vi "MAT_TestingVI.vi"() -> ()   [LabVIEW 2024]
uses:
  Subs/miDataType.ctl
panel:
  out "unsigned byte array":u8[](array[numeric])
  out "dimensions":i32[](array[numeric])
  out "Arrays same?":bool
  out "Matrix":T2
  out "Waveform Graph":i16[](graph)
  out "unsigned byte array 2":u8[](array[numeric])
  out "mine":u8[](array[numeric]) format="%.0b"
  out "Bytes same?":bool
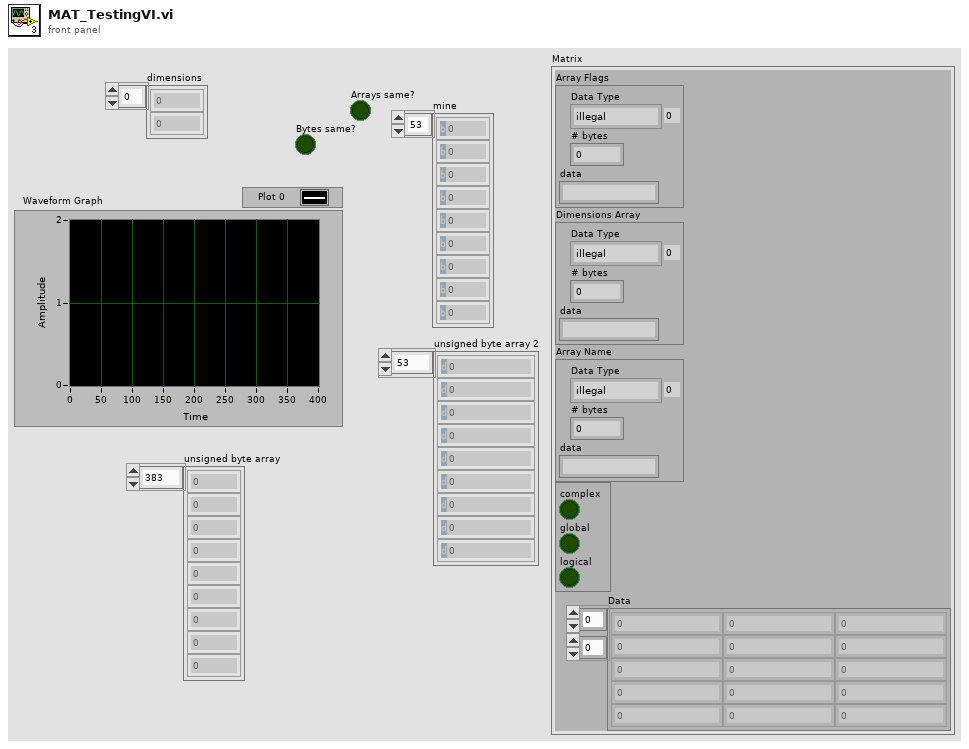
[diagram p1: front panel]
types:
  T1 = typedef "miDataType.ctl" = enum16{"illegal", "miINT8", "miUINT8", "miINT16", "miUINT16", "miINT32", "miUINT32", "miSINGLE", "--", "miDOUBLE", "---", "----", "miINT64", "miUINT64", "miMATRIX", "miCOMPRESSED", "miUTF8", "miUTF16", "miUTF32", "udefined"}
  T2 = cluster{"Array Flags":cluster{"Data Type":T1, "# bytes":u32, "data":string}, "Dimensions Array":cluster{"Data Type":T1, "# bytes":u32, "data":string}, "Array Name":cluster{"Data Type":T1, "# bytes":u32, "data":string}, cluster{"complex":bool, "global":bool, "logical":bool}, "Data":dbl[][]}
  T3 = enum16{"big-endian, network order", "native, host order", "little-endian"}
  T4 = cluster{"Data Type":T1, "# bytes":u32, "data":string}
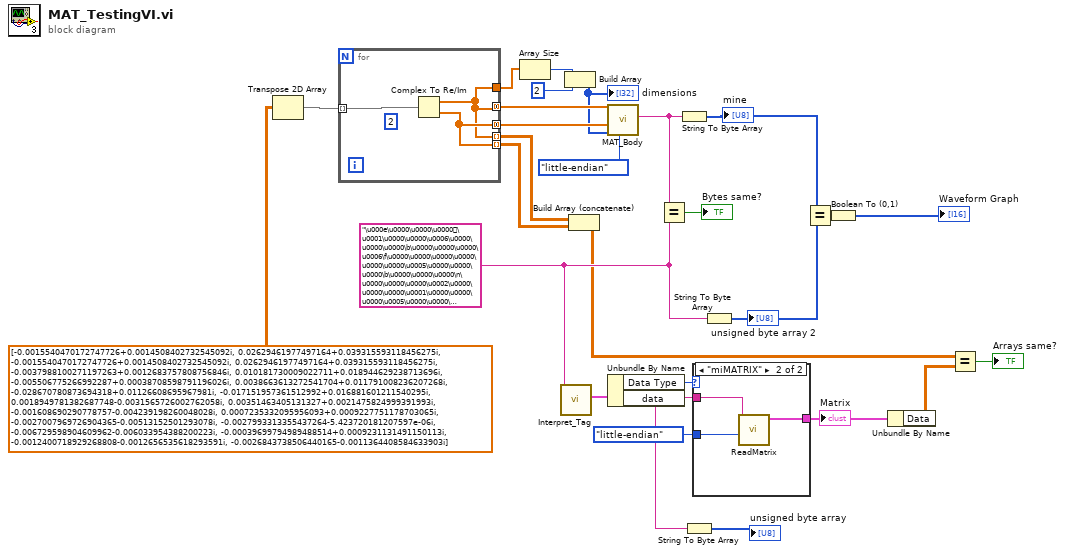
[diagram p0: block diagram]
diagram:
  w17 = "\u000e\u0000\u0000\u0000\u0001\u0000\u0000\u0006\u0000\u0000\u0000\b\u0000\u0000\u0000\u0006\f\u0000\u0000\u0000\u0000\u0000\u0000\u0005\u0000\u0000\u0000\b\u0000\u0000\u0000\n\u0000\u0000\u0000\u0002\u0000\u0000\u0000\u0001\u0000\u0000\u0000\u0005\u0000\u0000\u0000yspec\u0000\u0000\u0000\t\u0000\u0000\u0000 \u0000\u0000\u0000«fG%vY¿«fG%vY¿h÷®\u001eo¿·ÙºEv¿¸-Ðß[¿ö\u0019ZH\u001d\f_?ûæ\f\fV[Z¿\u0007wUû\u001ff¿S2^ó~{¿Hc\u000e=QT¿Ê\u001eú\u000fúì?Ê\u001eú\u000fúì?×^>«(Ú?(ûîX¬o?#h¸_H¿3|ÙÉ¸Êl?¸'¼oµG?²-îf¿J×\u001c6\u0004:¿þÂ<ýe¿\t\u0000\u0000\u0000 \u0000\u0000\u0000wLáCÅW?wLáCÅW?ûÝ\u001fôÇT?P¨¨9^9?Ì ]¬\u0012?­½\u0002ÐÛi¿ôí5\u001e\u001f]q¿q\r¿AË\u0004u¿\u0018½4L\u000f·x¿_ëý)¼T¿7NUe,!¤?7NUe,!¤?Í{\u000f8f?ÀL\u0017Vâ%?Cn\u0014iI?'SIÎa?ÓÛõyÌ<N?1ìÙ¬¿Ö¾\\9d¢?N?SA\u0014R¿"
  n1 = Transpose 2D Array(2D array=cdb[][] [[-0.0015540470172747726+0.0014508402732545092i, 0.02629461977497164+0.039315593118456275i], [-0.0015540470172747726+0.0014508402732545092i, 0.02629461977497164+0.039315593118456275i], [-0.0037988100271197263+0.0012683757808756846i, 0.010181730009022711+0.018944629238713696i], [-0.005506775266992287+0.00038708598791196026i, 0.0038663613272541704+0.011791008236207268i], [-0.028670780873694318+0.01126608695967981i, -0.017151957361512992+0.016881601211540295i], [0.0018949781382687748-0.0031565726002762058i, 0.00351463405131327+0.0021475824999391993i], [-0.001608690290778757-0.004239198260048028i, 0.0007235332095956093+0.0009227751178703065i], [-0.0027007969726904365-0.00513152501293078i, -0.0027993313355437264-5.423720181207597e-06i], [-0.006729598904609962-0.006033954388200223i, -0.00039699794989488514+0.0009231131491150113i], [-0.0012400718929268808-0.0012656535618293591i, -0.0026843738506440165-0.0011364408584633903i]] ("complex")) -> (transposed array=w20:cdb[][])
  n2 = for {
    tunnel: w20 -> [w30] mode=indexing
    tunnel: [w28] -> w11 mode=concatenating
    tunnel: [w29] -> w14 mode=concatenating
    tunnel: [w28] -> w7 mode=indexing
    tunnel: [w29] -> w6 mode=indexing
    tunnel: [w28] -> w8
    (unwired) 2 ("index")
    n3 = Complex To Re/Im(x + iy=w30) -> (x=w28:dbl[], y=w29:dbl[])
  }
  n4 = Array Size(array=w8) -> (size(s)=w3:i32)
  n5 = call "Interpret_Tag.vi"("String in"=w17) -> ("Tag"=w19:T4)  [unwired: 8 in, 2 out]
  n6 = Build Array(w3, 2 ("index")) -> (w1:i32[])
  "dimensions" <- w1
  n7 = Build Array (concatenate)(w7, w6) -> (w13:dbl[][])
  n8 = call "MAT_Body.vi"("byte order"=T3."little-endian", "Dimensions"=w1, "Imag"=w14, "Real"=w11) -> ("String Out"=w25:string)  [unwired: 6 in, 1 out]
  n9 = Unbundle By Name(w19) -> ("Data Type"=w18:T1, "data"=w4:string)
  n10 = Equal?(x=w25, y=w17) -> (x = y?=→"Bytes same?":bool)
  n11 = String To Byte Array(string=w25) -> (unsigned byte array=w24:u8[])
  "mine" <- w24
  n12 = String To Byte Array(string=w4) -> (unsigned byte array=→"unsigned byte array":u8[])
  n13 = case shown="\"miMATRIX\"" w18 {
    tunnel: w4 -> [_ w33]
    tunnel: [_ w31] -> w15
    tunnel: T3."little-endian" ("Endian") -> [_ w32]
    frame Default {
    }
    frame "miMATRIX" {
      n14 = call "ReadMatrix.vi"("byte order"=w32, "String in"=w33) -> ("Matrix"=w31:T2)  [unwired: 6 in, 3 out]
    }
  }
  "Matrix" <- w15
  n15 = String To Byte Array(string=w17) -> (unsigned byte array=w21:u8[])
  "unsigned byte array 2" <- w21
  n16 = Equal?(x=w24, y=w21) -> (x = y?=w23:bool[])
  n17 = Boolean To (0,1)(Boolean=w23) -> (0, 1=→"Waveform Graph":i16[])
  n18 = Unbundle By Name(w15) -> ("Data"=w10:dbl[][])
  n19 = Equal?(x=w13, y=w10) -> (x = y?=→"Arrays same?":bool)
